vi "Initialize.vi"(8 "error in (no error)":errorcluster, 11 "VISA in":refnum<class "VISA.lvclass">) -> (0 "error out":errorcluster, 3 "VISA out":refnum<class "VISA.lvclass">)   [LabVIEW 2019, in "Protocols.lvlib" / "VISA.lvclass"]
uses:
  VISA.lvclass
  VISA.lvclass/VISA.ctl
  Data Access/Read VISA Resource.vi
  Data Access/Read Timeout.vi
  Data Access/Read Enable Termination Character.vi
  Data Access/Read Termination Character.vi
  Data Access/Write Ref.vi
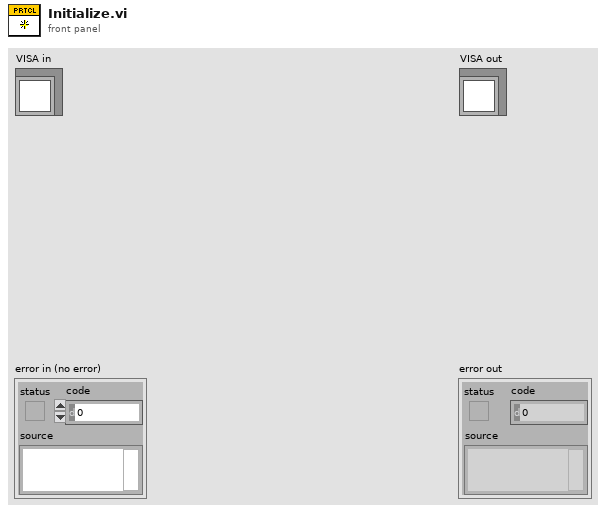
[diagram p1: front panel]
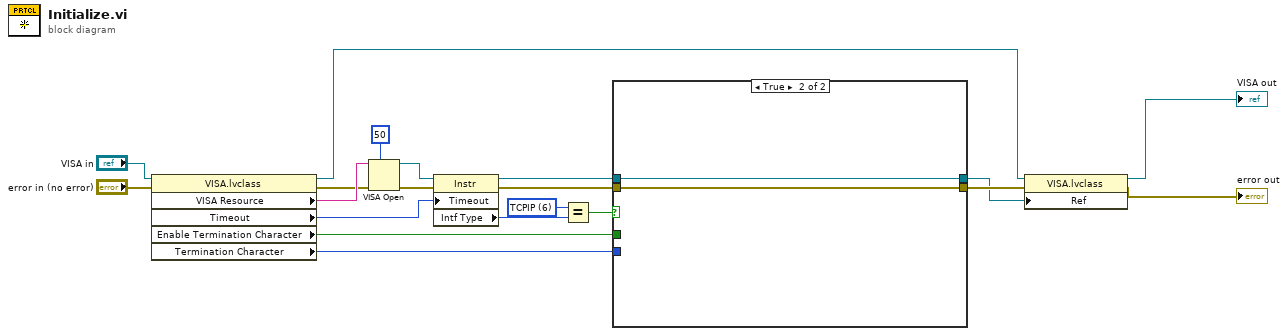
[diagram p0: block diagram]
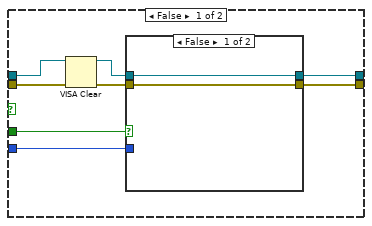
[diagram p2: hidden frame]
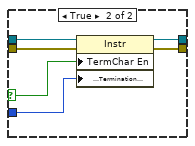
[diagram p3: hidden frame]
diagram:
  w2 = u16 6 items=["GPIB"=1, "VXI"=2, "GPIB-VXI"=3, "Serial"=4, "PXI"=5, "TCPIP"=6, "USB"=7] ("Interface Information:Interface Type")
  n1 = property class="VISA.lvclass"(reference="VISA in", error in="error in (no error)") -> (reference out=w17:refnum<class "VISA.lvclass">, error out=w18:errorcluster, "VISA Resource"=w20:string, "Timeout"=w8:u32, "Enable Termination Character"=w14:bool, "Termination Character"=w13:u8)
  n2 = VISA Open(timeout (0)=u32 50 ("VISA Open timeout (0)"), error in (no error)=w18, VISA resource name=w20) -> (VISA resource name=w5:refnum<visa-resource-name>, error out=w7:errorcluster)  [unwired: 2 in]
  n3 = property class="Instr"(reference=w5, error in=w7, "Timeout"=w8) -> (reference out=w4:refnum<visa-resource-name>, error out=w6:errorcluster, "Intf Type"=w3:u16)
  n4 = Equal?(x=w2, y=w3) -> (x = y?=w1:bool)
  n5 = case shown="True" w1 {
    tunnel: w14 -> [w26 _]
    tunnel: w13 -> [w25 _]
    tunnel: [w24 w37] -> w10
    tunnel: [w23 w38] -> w9
    tunnel: w6 -> [w22 w37]
    tunnel: w4 -> [w21 w38]
    frame False {
      n6 = VISA Clear(VISA resource name=w21, error in (no error)=w22) -> (VISA resource name out=w27:refnum<visa-resource-name>, error out=w28:errorcluster)
      n7 = case shown="False" w26 {
        selector: w26 -> [_ w31]
        tunnel: w27 -> [w29 w36]
        tunnel: w28 -> [w30 w35]
        tunnel: [w29 w34] -> w23
        tunnel: [w30 w33] -> w24
        tunnel: w25 -> [_ w32]
        frame False {
        }
        frame True {
          n8 = property class="Instr"(reference=w36, error in=w35, "TermChar En"=w31, "Message Based Settings:Termination Character"=w32) -> (reference out=w34:refnum<visa-resource-name>, error out=w33:errorcluster)
        }
      }
    }
    frame True {
    }
  }
  n9 = property class="VISA.lvclass"(reference=w17, error in=w10, "Ref"=w9) -> (reference out=→"VISA out":refnum<class "VISA.lvclass">, error out=→"error out":errorcluster)
